vi "Read Variant Data.vi"(8 "error in (no error)":errorcluster, 11 "My Custom Type in":refnum<class "My Custom Type.lvclass">) -> (0 "error out":errorcluster, 2 "data":variant, 3 "My Custom Type out":refnum<class "My Custom Type.lvclass">)   [LabVIEW 2020, in "My Custom Type.lvclass"]
uses:
  My Custom Type.lvclass
  My Custom Type.lvclass/My Custom Type.ctl
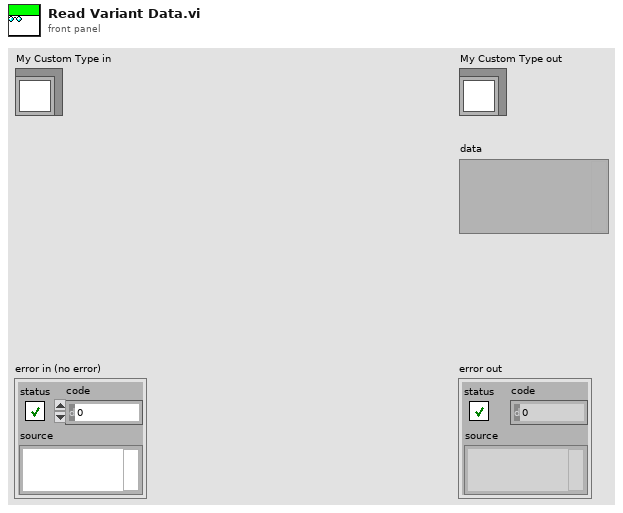
[diagram p1: front panel]
types:
  T1 = typedef "Custom Structure.ctl" = cluster{"timeStamp":T2, "fieldB":string, "fieldA":i32, "fieldC":cluster{"fieldC1":bool, "fieldC2":dbl}}
  T2 = typedef "PV Access.lvlib/PV Data.lvlib/EPICS Timestamp.ctl" = cluster{"secondsPastEpoch":i64, "nanoseconds":i32, "userTag":i32}
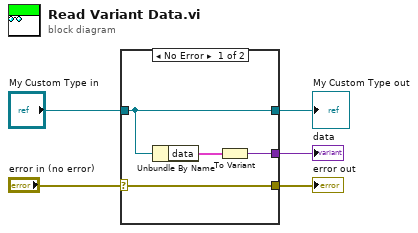
[diagram p0: block diagram]
diagram:
  n1 = case shown="No Error" "error in (no error)" {
    selector: "error in (no error)" -> [w8 w10]
    tunnel: [w6 _] -> w5
    tunnel: "My Custom Type in" -> [w9 w11]
    tunnel: [w9 w11] -> w3
    tunnel: [w8 w10] -> w1
    frame No Error {
      n2 = Unbundle By Name(w9) -> ("data"=w7:T1)
      n3 = To Variant(anything=w7) -> (Variant=w6:variant)
    }
    frame Error {
    }
  }
  "error out" <- w1
  "My Custom Type out" <- w3
  "data" <- w5
